vi "Ejemplo de limit switch.vi"() -> ()   [LabVIEW 2014]
uses:
  <vilib>/Rock Robotics/SystemInterfaces/DIO/FPGA_DIOChannel.ctl
  <vilib>/Rock Robotics/WPI/Switch/WPI_SwitchOpenLimit.vi
panel:
  out "#pressed":i32
  out "Pressed?":bool
  in  "DIO Channel":T1
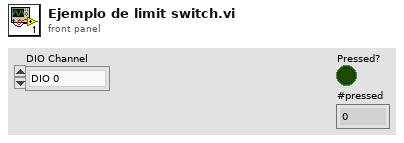
[diagram p1: front panel]
types:
  T1 = typedef "FPGA_DIOChannel.ctl" = enum8{"DIO 0", "DIO 1", "DIO 2", "DIO 3", "DIO 4", "DIO 5", "DIO 6", "DIO 7", "DIO 8", "DIO 9", "DIO MXP 0", "DIO MXP 1", "DIO MXP 2", "DIO MXP 3", "DIO MXP 4", "DIO MXP 5", "DIO MXP 6", "DIO MXP 7", "DIO MXP 8", "DIO MXP 9", "DIO MXP 10", "DIO MXP 11", "DIO MXP 12", "DIO MXP 13", "DIO MXP 14", "DIO MXP 15", "Invalid"}
  T2 = typedef "WPI_SwitchDevRef.ctl" = cluster{"DevStatus":errorcluster, "DIO Channel":T1, "Controller":T3, "CntIndex":T4, "Normally Closed":bool}
  T3 = typedef "FPGA_TypedefDigitalModule.ctl" = enum16{"Controller 1"}
  T4 = typedef "FPGA_CounterCtrSystemIndex.ctl" = enum8{"Ctr 0", "Ctr 1", "Ctr 2", "Ctr 3", "Ctr 4", "Ctr 5", "Ctr 6", "Ctr 7", "Invalid"}
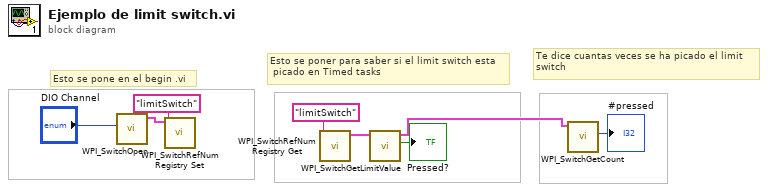
[diagram p0: block diagram]
diagram:
  # "Te dice cuantas veces se ha picado el limit\nswitch"
  # "Esto se poner para saber si el limit switch esta\n picado en Timed tasks"
  # "Esto se pone en el begin .vi"
  n1 = call-poly <vilib>:"WPI_SwitchOpen.vi"("DIO Channel"="DIO Channel") -> ("SwitchDevRef"=w7:T2)  [unwired: 9 in, 1 out]
  n2 = call <vilib>:"WPI_SwitchRefNum Registry Set.vi"("refnum name"="limitSwitch", "SwitchDevRef"=w7) -> ()  [unwired: 8 in, 2 out]
  n3 = call <vilib>:"WPI_SwitchRefNum Registry Get.vi"("refnum name"="limitSwitch") -> ("SwitchDevRef"=w6:T2)  [unwired: 9 in, 1 out]
  n4 = call <vilib>:"WPI_SwitchGetLimitValue.vi"("SwitchDevRef"=w6) -> ("Switch Pressed"=→"Pressed?":bool, "SwitchDevRef"=w2:T2)  [unwired: 8 in, 1 out]
  n5 = call <vilib>:"WPI_SwitchGetCount.vi"("SwitchDevRef"=w2) -> ("Switch Pressed Count"=→"#pressed":i32)  [unwired: 8 in, 2 out]
